vi "SMC_AxisAbs.vi"(8 "error in (no error)":errorcluster, 9 "WaitUntilReady":bool, 10 "Distance":dbl format="%.6f", 11 "AxisNr":u8) -> (0 "error out":errorcluster)   [LabVIEW 2015]
doc: "AxisNr is only used in VENUS 1. It is ignored in VENUS 2"
uses:
  SMC_SubVIs.llb/SMC_ManagerMode.ctl
  SMC_SubVIs.llb/glb_stop.vi
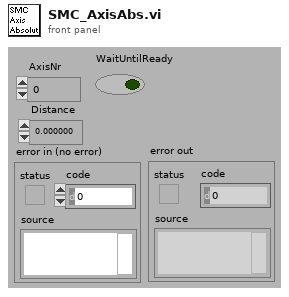
[diagram p1: front panel]
types:
  T1 = typedef "SMC_ManagerMode.ctl" = enum16{"Init", "Get", "SetPosition", "SetStatus", "SetMoving", "SetControllerNr"}
  T2 = typedef "SMC Paras.ctl" = cluster{"VENUS Language":T3, "Number of Axis":u8, "Controller Nr":u8, "Simulation":bool}
  T3 = typedef "VENUSNr.ctl" = enum16{"VENUS 2", "VENUS 1"}
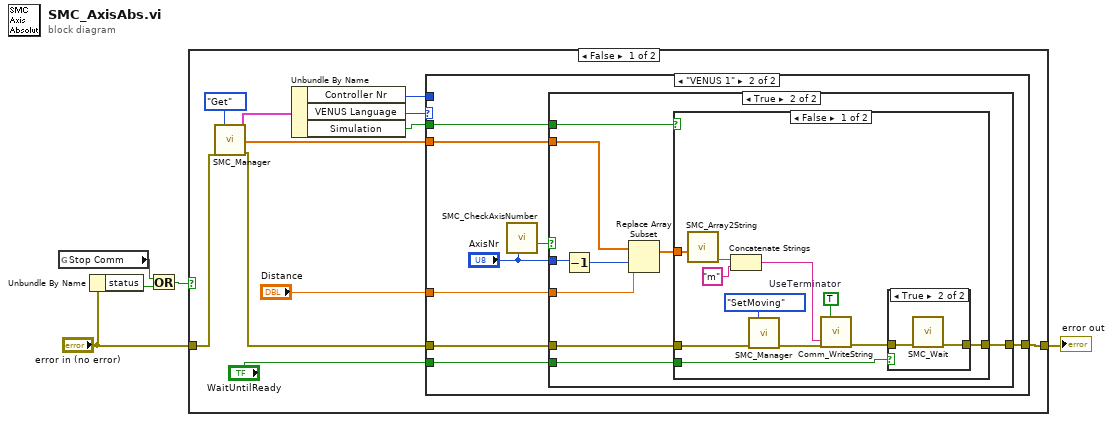
[diagram p0: block diagram]
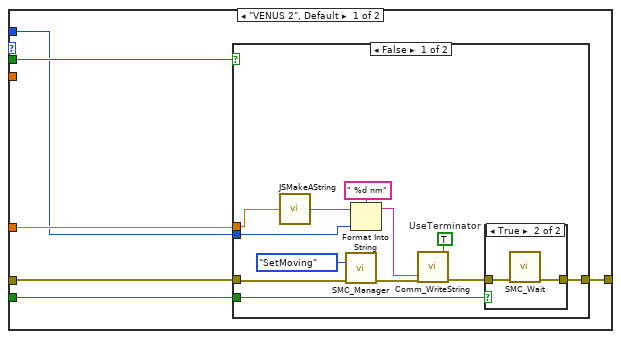
[diagram p2: hidden frame]
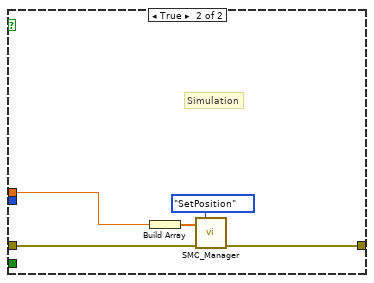
[diagram p4: hidden frame]
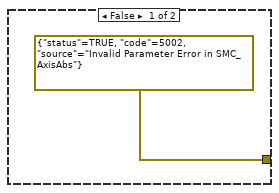
[diagram p5: hidden frame]
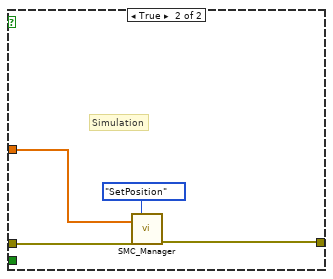
[diagram p7: hidden frame]
diagram:
  n1 = global read "glb_stop.vi" "Stop Comm"() -> (w1:bool)
  n2 = Unbundle By Name("error in (no error)") -> ("status"=w5:bool)
  n3 = Or(x=w1, y=w5) -> (x .or. y?=w2:bool)
  n4 = case shown="False" w2 {
    tunnel: "error in (no error)" -> [w15 w79]
    tunnel: [w14 w79] -> w3
    frame False {
      n5 = call "SMC_Manager.vi"("Mode"=SMC_ManagerMode."Get", "error in (no error)"=w15) -> ("SMC Parameter Out"=w9:T2, "Position"=w12:dbl[], "error out"=w13:errorcluster)  [unwired: 9 in, 2 out]
      n6 = Unbundle By Name(w9) -> ("Controller Nr"=w7:u8, "VENUS Language"=w8:T3, "Simulation"=w6:bool)
      n7 = case shown="\"VENUS 1\"" w8 {
        tunnel: [w20 w48] -> w14
        tunnel: w13 -> [w21 w47]
        tunnel: w6 -> [w22 w46]
        tunnel: w12 -> [_ w45]
        tunnel: "Distance" -> [w18 w44]
        tunnel: "WaitUntilReady" -> [w19 w43]
        tunnel: w7 -> [w17 _]
        frame "VENUS 2", Default {
          n8 = case shown="False" w22 {
            tunnel: w21 -> [w30 w41]
            tunnel: [w26 w40] -> w20
            tunnel: w19 -> [w31 _]
            tunnel: w18 -> [w25 w38]
            tunnel: w17 -> [w27 _]
            frame False {
              w23 = TRUE  # UseTerminator
              n9 = call "JSMakeAString.vi"("Value"=w25) -> ("String"=w24:string)
              n10 = call "SMC_Manager.vi"("Mode"=SMC_ManagerMode."SetMoving", "error in (no error)"=w30) -> ("error out"=w33:errorcluster)  [unwired: 9 in, 4 out]
              n11 = Format Into String(format string=" %d nm" ("Format String"), initial string=w24, w27) -> (resulting string=w28:string)  [unwired: 1 in, 1 out]
              n12 = call "Comm_WriteString.vi"("string to write"=w28, "error in (no error)"=w33, "UseTerminator"=w23) -> ("error out"=w32:errorcluster)  [unwired: 8 in]
              n13 = case shown="True" w31 {
                tunnel: w32 -> [w35 w37]
                tunnel: [w35 w36] -> w26
                frame False {
                }
                frame True {
                  n14 = call "SMC_Wait.vi"("error in (no error)"=w37) -> ("error out"=w36:errorcluster)  [unwired: 10 in]
                }
              }
            }
            frame True {
              # "Simulation"
              n15 = Build Array(w38) -> (w39:dbl[])
              n16 = call "SMC_Manager.vi"("Mode"=SMC_ManagerMode."SetPosition", "PosArraySimu"=w39, "error in (no error)"=w41) -> ("error out"=w40:errorcluster)  [unwired: 8 in, 4 out]
            }
          }
        }
        frame "VENUS 1" {
          n17 = call "SMC_CheckAxisNumber.vi"("AxisNr"="AxisNr") -> ("Result"=w50:bool)  [unwired: 10 in]
          n18 = case shown="True" w50 {
            tunnel: w45 -> [_ w58]
            tunnel: "AxisNr" -> [_ w57]
            tunnel: w47 -> [_ w55]
            tunnel: [errorcluster {"status"=TRUE, "code"=5002, "source"="Invalid Parameter Error in SMC_AxisAbs"} ("t") w56] -> w48
            tunnel: w46 -> [_ w54]
            tunnel: w44 -> [_ w53]
            tunnel: w43 -> [_ w52]
            frame False {
            }
            frame True {
              n19 = Decrement(x=w57) -> (x-1=w59:u8)
              n20 = Replace Array Subset(array=w58, new element=w53, index=w59) -> (w60:dbl[])
              n21 = case shown="False" w54 {
                tunnel: w60 -> [w66 w75]
                tunnel: [w63 w77] -> w56
                tunnel: w55 -> [w67 w78]
                tunnel: w52 -> [w62 _]
                frame False {
                  w61 = TRUE  # UseTerminator
                  n22 = call "SMC_Array2String.vi"("Input Array"=w66) -> ("String"=w65:string)  [unwired: 10 in]
                  n23 = Concatenate Strings(w65, "m" ("Substring")) -> (w70:string)
                  n24 = call "SMC_Manager.vi"("Mode"=SMC_ManagerMode."SetMoving", "error in (no error)"=w67) -> ("error out"=w68:errorcluster)  [unwired: 9 in, 4 out]
                  n25 = call "Comm_WriteString.vi"("string to write"=w70, "error in (no error)"=w68, "UseTerminator"=w61) -> ("error out"=w64:errorcluster)  [unwired: 8 in]
                  n26 = case shown="True" w62 {
                    tunnel: w64 -> [w72 w74]
                    tunnel: [w72 w73] -> w63
                    frame False {
                    }
                    frame True {
                      n27 = call "SMC_Wait.vi"("error in (no error)"=w74) -> ("error out"=w73:errorcluster)  [unwired: 10 in]
                    }
                  }
                }
                frame True {
                  # "Simulation"
                  n28 = call "SMC_Manager.vi"("Mode"=SMC_ManagerMode."SetPosition", "PosArraySimu"=w75, "error in (no error)"=w78) -> ("error out"=w77:errorcluster)  [unwired: 8 in, 4 out]
                }
              }
            }
          }
        }
      }
    }
    frame True {
      # "Error, do nothing"
    }
  }
  "error out" <- w3
